vi "12.简单事件触发.vi"() -> ()   [LabVIEW 2019]
uses:
  <vilib>/Platform/TimedLoop/XDataNode/timing_clust.ctl
  <vilib>/Platform/TimedLoop/XDataNode/nitl_modes.ctl
  <vilib>/Platform/TimedLoop/XDataNode/wakeup.ctl
  <vilib>/rvi/Emulation/niFpgaGetClockAttributes.vi
  <vilib>/rvi/Emulation/niFpgaSctlEmulationGetInTimedLoop.vi
  <vilib>/rvi/Emulation/niFpgaEmulationReportErrorSimple.vi
  <vilib>/rvi/Emulation/niFpgaCriticalErrorInLSC.vi
  <vilib>/rvi/eio/common/nirviEmuTemplateMethod_errors.vi
  <vilib>/Platform/TimedLoop/XDataNode/XDataNode.xnode
  <vilib>/eio/EIONode/EIONode.xnode
  <vilib>/Platform/TimedLoop/XDataNode/XDNodeRunTimeDep.lvlib
panel:
  in  "ConnectorA/AO0":sgl(slide) scale=1.0..5.0
  in  "Count(uSec)":u16=100 caption="计数器(uSec)"
  out "ConnectorA/AI0":fxp<+/-,24,5>
  in  "阈值":fxp<+/-,24,5>=3.0
  out "布尔":bool
  in  "Count(uSec) 2":u16=10 caption="计数器(uSec)"
  in  "采样点数":i32=300000
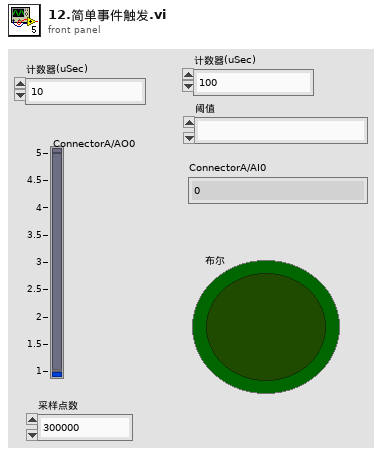
[diagram p1: front panel]
types:
  T1 = typedef "XDNodeRunTimeDep.lvlib/timing_clust.ctl" = cluster{"Expected End [f-1]":u64, "Actual End [f-1]":u64, "Finished Late? [f-1]":bool, "Expected End [i-1]":u64, "Actual End [i-1]":u64, "Finished Late? [i-1]":bool, "Expected Start [i]":u64, "Actual Start [i]":u64, "Expected Start [f]":u64, "Actual Start [f]":u64, "Source Name":string, "Structure Name":string, "Period":i64, "Deadline":i64, "Offset":i64, "Start":i64, "Priority":i32, "Timeout":i32, "Mode":T2, "Wakeup Reason":T3, "Error":errorcluster, "Source Type":string, "Secondary Source Type":string, "Global End Time":u64, "Global Start Time":u64, "Frame Duration":u64, "Iteration Duration":u64, "Assigned CPU":i32, "I/O Scan Engine Mode":u32}
  T2 = typedef "XDNodeRunTimeDep.lvlib/nitl_modes.ctl" = enum32{"No Change", "Process missed periods, maintain original phase", "Discard missed periods, maintain original phase", "Process missed periods, ignore original phase", "Discard missed periods, ignore original phase"}
  T3 = typedef "XDNodeRunTimeDep.lvlib/wakeup.ctl" = enum32{"Normal", "Aborted", "Asynchronous wakeup", "Timing source error", "Timed loop error", "Timeout"}
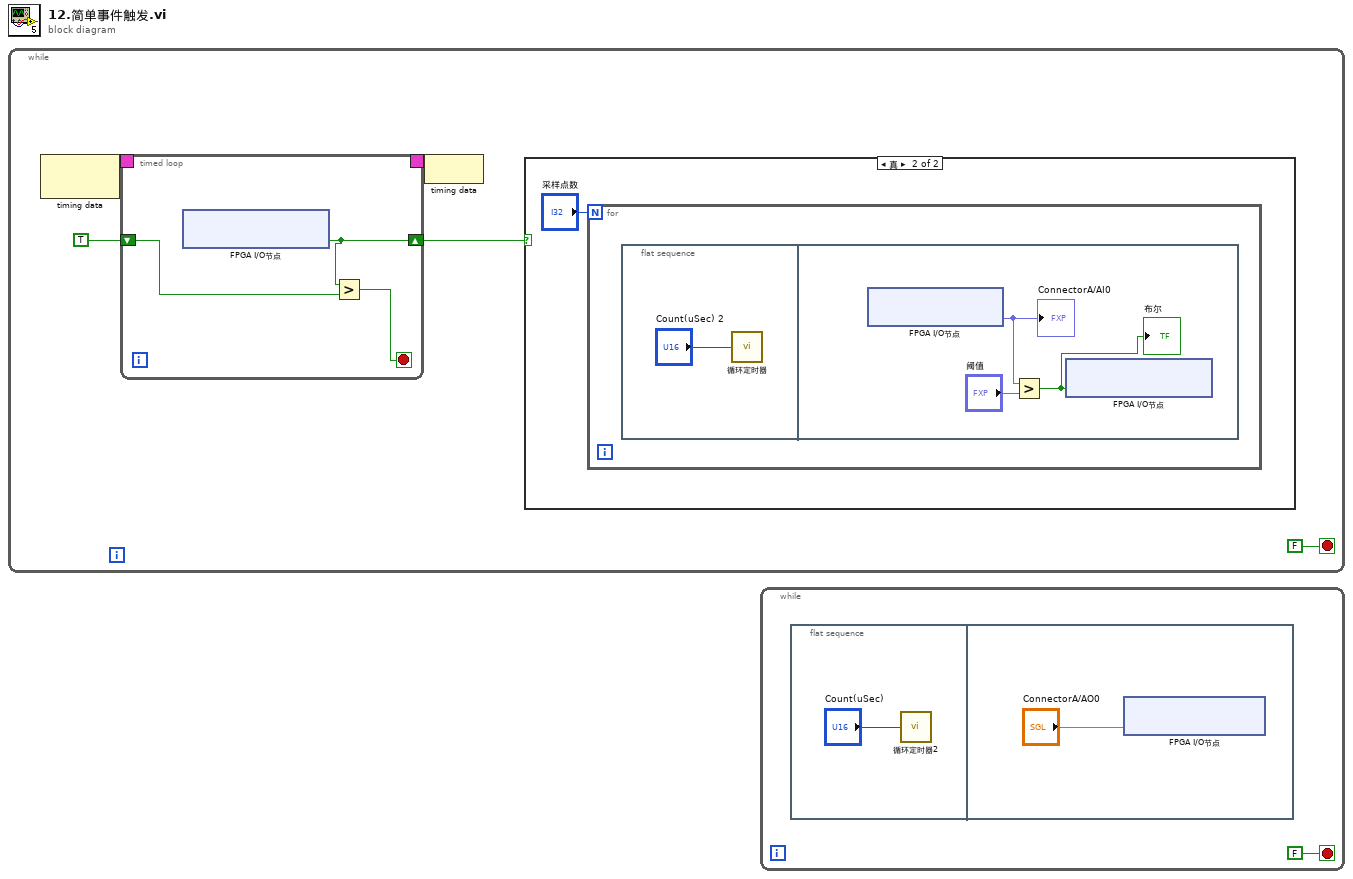
[diagram p0: block diagram]
diagram:
  n1 = while {
    stop <- FALSE stop-if-true
    n2 = node-c288() -> (w4:T1)  [unwired: 1 in]
    n3 = timed-loop {
      timing: w4 -> [_]
      timing-out: [_] -> w3
      shift-right: [w8] -> w1
      shift-left: TRUE -> [w7]
      stop <- w6 stop-if-true
      n4 = xnode "FPGA I/O节点"() -> ("ConnectorA/DIO1"=w8:bool)  [unwired: 1 in, 1 out]
      n5 = Greater?(x=w8, y=w7) -> (0:w6:bool)
    }
    n6 = node-c288(w3) -> ()
    n7 = case shown="真" w1 {
      frame False {
      }
      frame True {
        n8 = for {
          N: "采样点数" -> [_]
          n9 = flat-sequence {
            frame #0 {
              n10 = call "循环定时器"("Count(uSec)"="Count(uSec) 2") -> ()  [unwired: 1 out]
            }
            frame #1 {
              n11 = xnode "FPGA I/O节点"() -> ("ConnectorA/AI0"=w17:fxp<+/-,24,5>)  [unwired: 1 in, 1 out]
              "ConnectorA/AI0" <- w17
              n12 = Greater?(x=w17, y="阈值") -> (0:w15:bool)
              "布尔" <- w15
              n13 = xnode "FPGA I/O节点"("ConnectorA/DIO0"=w15) -> ()  [unwired: 1 in, 1 out]
            }
          }
        }
      }
    }
  }
  n14 = while {
    stop <- FALSE stop-if-true
    n15 = flat-sequence {
      frame #0 {
        n16 = call "循环定时器2"("Count(uSec)"="Count(uSec)") -> ()  [unwired: 1 out]
      }
      frame #1 {
        n17 = xnode "FPGA I/O节点"("ConnectorA/AO0"="ConnectorA/AO0") -> ()  [unwired: 1 in, 1 out]
      }
    }
  }
